vi "dscommands.vi"() -> ()   [LabVIEW 2019]
panel:
  out "Pre_Spin":bool
  out "DS_Shooter_Triggers":bool[](array[boolean])
  out "Clear_Jams":bool
  out "Master_State_Triggers":bool[](array[boolean])
  out "Driver_RightTrigger":dbl
  out "Driver_RightY":dbl
  out "Driver_RightX":dbl
  out "Driver_LeftX":dbl
  out "Driver_LeftTrigger":dbl
  out "Driver_LeftY":dbl
  out "Driver_RightTriggerBoolean":bool
  out "Driver_LeftTriggerBoolean":bool
  out "Driver_LeftJoystickButton":bool
  out "Driver_RightJoystickButton":bool
  out "Driver_RightBumper":bool
  out "Driver_LeftBumper":bool
  out "Driver_Menu":bool
  out "Driver_View":bool
  out "Driver_Y":bool
  out "Driver_X":bool
  out "Driver_B":bool
  out "Driver_A":bool
  # "--driver joystick--"
  # "--manipulator controls--"
  # "--autonomous controls--"
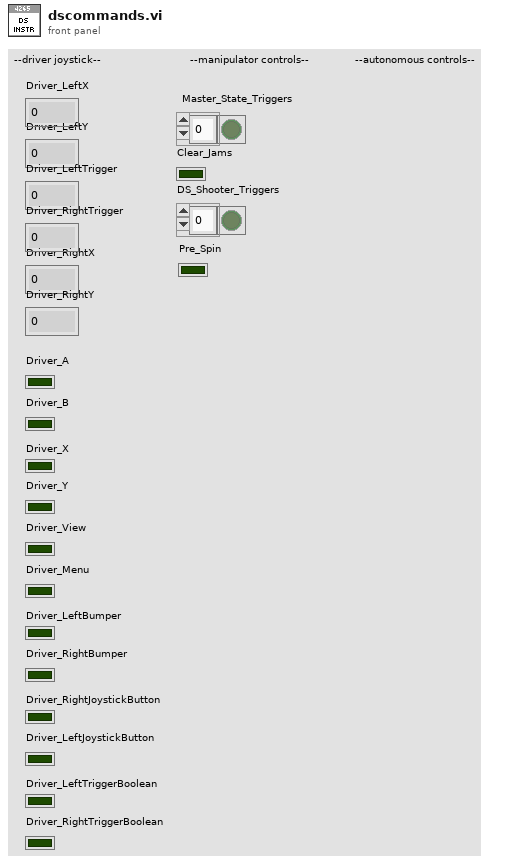
[diagram p1: front panel]
diagram:
